vi "R_W_Heater_Setup.vi"(2 "Mode":enum16{"Load from File", "Save to File"}(ring), 3 "Setpoints In":T1[](array[typedef])) -> (1 "Setpoints Out":T1[](array[typedef]))   [LabVIEW 2010]
uses:
  Heater_Setpoint.ctl
  Anemometry/Anemometry Sub Vis/File/Setup_Filetype.ctl
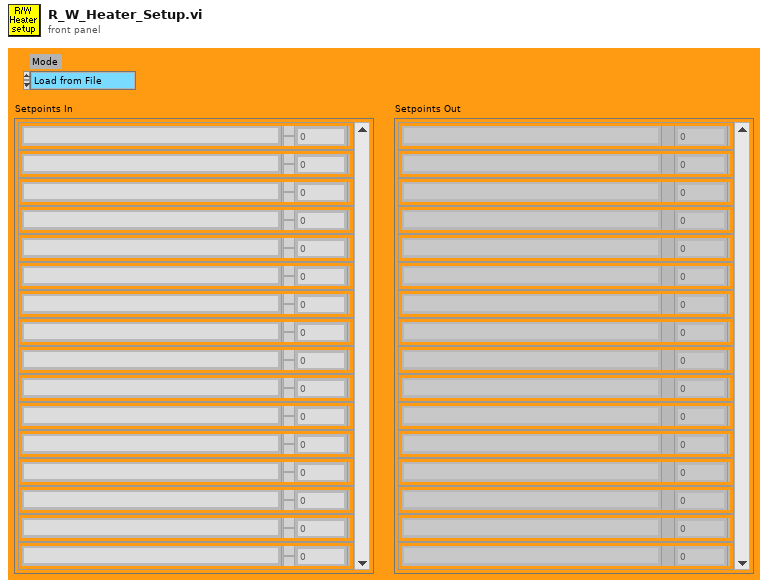
[diagram p1: front panel]
types:
  T1 = typedef "Heater_Setpoint.ctl" = cluster{"Ch Name":string, "Setpoint":dbl}
  T2 = typedef "Setup_Filetype.ctl" = enum16{"Measurement Setups", "Calibration Setups", "General", "Results File Plotter Setups", "Speed Calib Tweaks"}
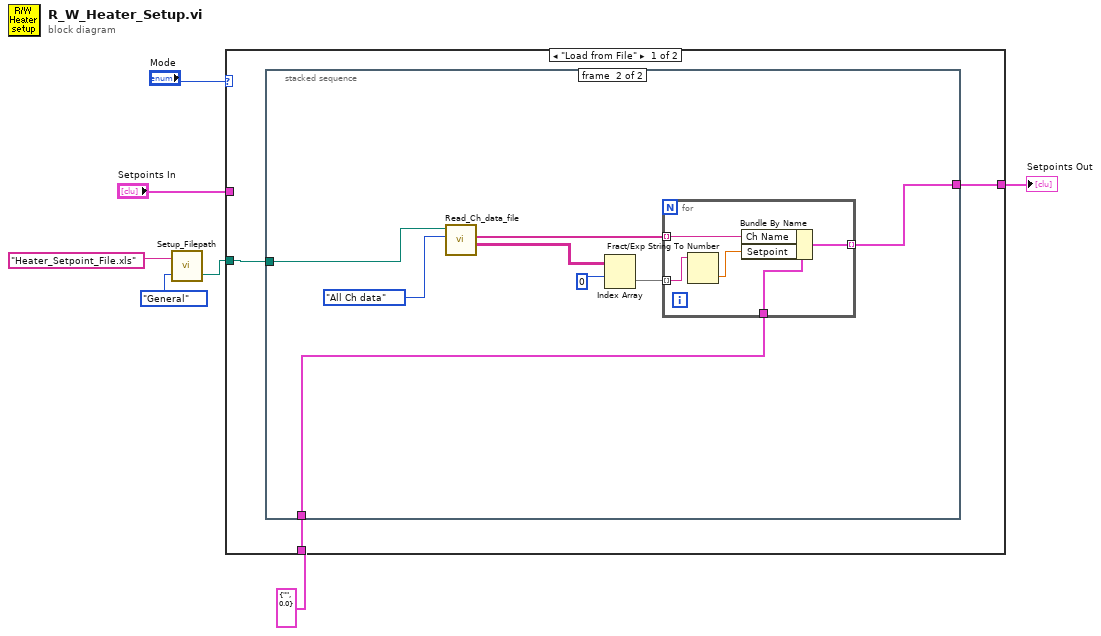
[diagram p0: block diagram]
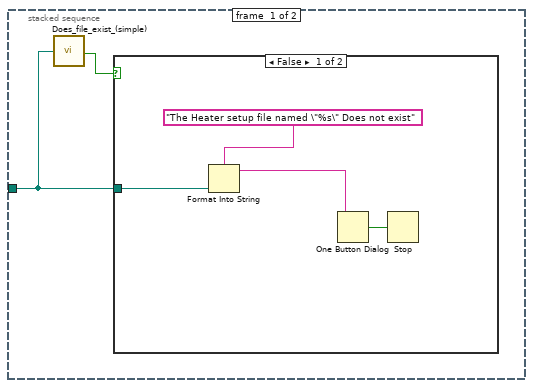
[diagram p2: hidden frame]
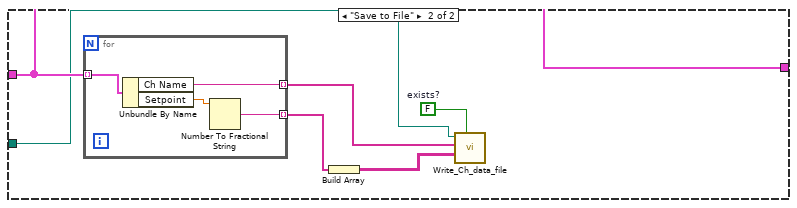
[diagram p4: hidden frame]
diagram:
  n1 = call "Setup_Filepath.vi"("Setup File Type"=Setup_Filetype."General", "Filename in"="Heater_Setpoint_File.xls" ("name or relative path")) -> ("Filename Out"=w1:path)  [unwired: 1 out]
  n2 = case shown="\"Load from File\"" "Mode" {
    tunnel: w1 -> [w8 w30]
    tunnel: T1 {"Ch Name"="", "Setpoint"=0.0} ("Cluster") -> [w10 _]
    tunnel: [w9 w31] -> w5
    tunnel: "Setpoints In" -> [_ w31]
    frame "Load from File" {
      n3 = stacked-sequence {
        tunnel: w8 -> [w11 w19]
        tunnel: w10 -> [_ w23]
        tunnel: [_ w21] -> w9
        frame #0 {
          n4 = call "Does_file_exist_(simple).vi"("Pathname"=w11) -> ("exists?"=w12:bool)
          n5 = case shown="False" w12 {
            tunnel: w11 -> [w16 _]
            frame False {
              n6 = Format Into String(format string="The Heater setup file named \"%s\" Does not exist" ("Format String"), w16) -> (resulting string=w15:string)  [unwired: 2 in, 1 out]
              n7 = One Button Dialog(message=w15) -> (true=w13:bool)  [unwired: 1 out]
              n8 = Stop(stop? (T)=w13) -> ()
            }
            frame True {
            }
          }
        }
        frame #1 {
          n9 = call "Read_Ch_data_file.vi"("Output"=enum16{"All Ch data", "The last few rows"}."All Ch data", "Filename"=w19) -> ("Channel Values"=w17:string[][], "Merged Channels"=w18:string[])  [unwired: 3 in, 3 out]
          n10 = Index Array(array=w17, index (row)=0 ("Index")) -> (element=w22:string[])  [unwired: 1 in]
          n11 = for {
            tunnel: w23 -> [w29]
            tunnel: w18 -> [w28] mode=indexing
            tunnel: w22 -> [w27] mode=indexing
            tunnel: [w25] -> w21 mode=indexing
            n12 = Fract/Exp String To Number(string=w27) -> (number=w26:dbl)  [unwired: 4 out]
            n13 = Bundle By Name(cluster=w29, "Ch Name"=w28, "Setpoint"=w26) -> (w25:T1)
          }
        }
      }
    }
    frame "Save to File" {
      w35 = FALSE  # exists?
      n14 = for {
        tunnel: w31 -> [w39] mode=indexing
        tunnel: [w37] -> w33 mode=indexing
        tunnel: [w36] -> w32 mode=indexing
        n15 = Unbundle By Name(w39) -> ("Ch Name"=w36:string, "Setpoint"=w38:dbl)
        n16 = Number To Fractional String(number=w38) -> (F-format string=w37:string)  [unwired: 3 out]
      }
      n17 = Build Array(w33) -> (w34:string[][])
      n18 = call "Write_Ch_data_file.vi"("exists?"=w35, "Channel Values"=w34, "Channel names"=w32, "Filename"=w30) -> ()  [unwired: 4 in, 4 out]
    }
  }
  "Setpoints Out" <- w5
